vi "backup.vi"(0 "dettes":dbl, 1 "Argent ventes":dbl, 2 "CA":dbl, 3 "Impots":dbl, 4 "Calculs button":bool) -> (5 "notions_cles":dbl[](array[numeric]))   [LabVIEW 2024]
uses:
  <vilib>/express/express shared/transition.llb/Dynamic To Waveform Array.vi
  <vilib>/express/express signal manip/GetorSetDDTAttributes/Set DDT Attributes/SetT0.vi
  <vilib>/express/express shared/transition.llb/Waveform Array To Dynamic.vi
  <vilib>/express/express signal manip/GetorSetDDTAttributes/Set DDT Attributes/Set DDT Properties.xnode
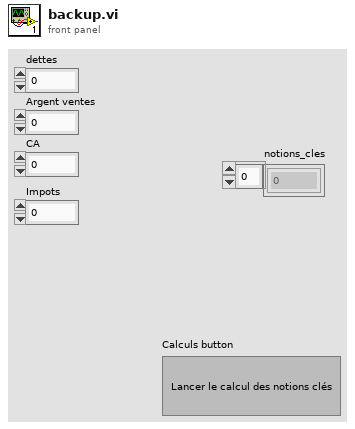
[diagram p1: front panel]
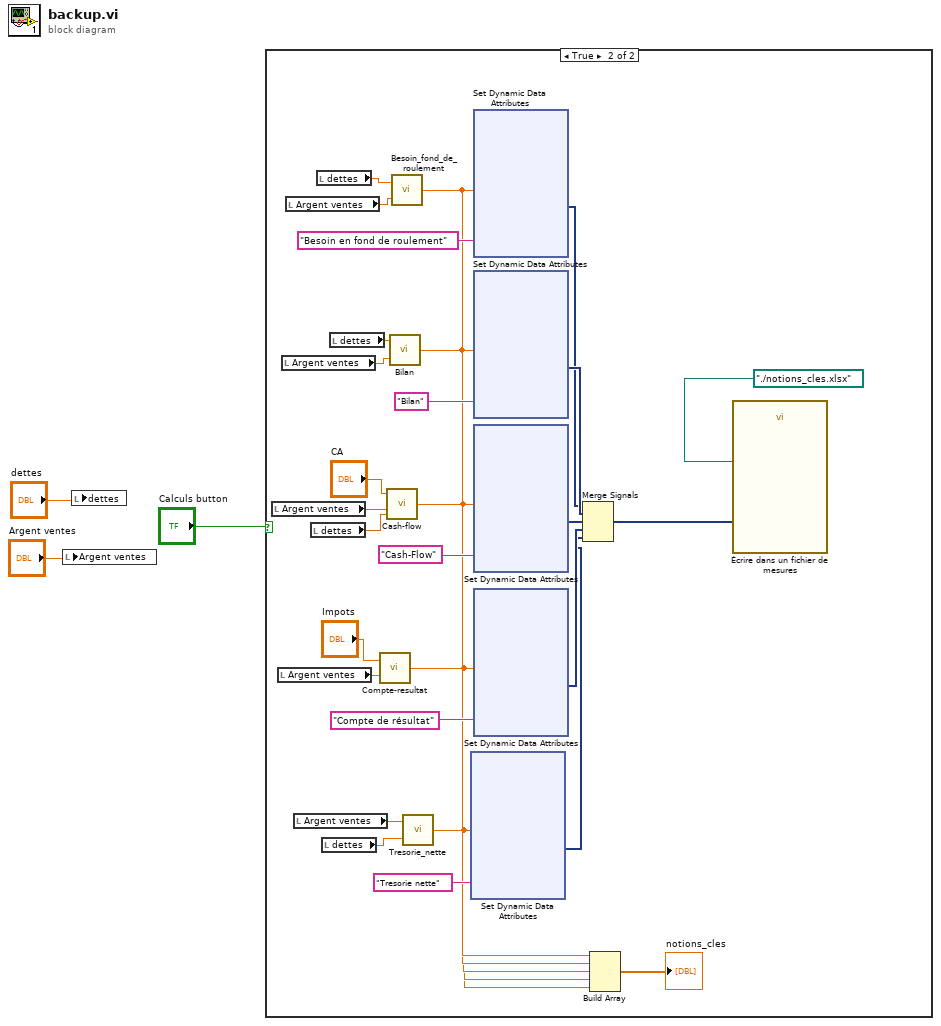
[diagram p0: block diagram]
diagram:
  n1 = local write "Argent ventes"("Argent ventes") -> ()
  n2 = local write "dettes"("dettes") -> ()
  n3 = case shown="True" "Calculs button" {
    frame False {
    }
    frame True {
      n4 = local read "Argent ventes"() -> (w16:dbl)
      n5 = local read "Argent ventes"() -> (w13:dbl)
      n6 = local read "Argent ventes"() -> (w18:dbl)
      n7 = local read "Argent ventes"() -> (w20:dbl)
      n8 = local read "Argent ventes"() -> (w12:dbl)
      n9 = local read "dettes"() -> (w15:dbl)
      n10 = local read "dettes"() -> (w21:dbl)
      n11 = local read "dettes"() -> (w11:dbl)
      n12 = local read "dettes"() -> (w19:dbl)
      n13 = call "Compte-resultat.vi"("Argent ventes"=w13, "Impots"="Impots") -> ("Compte résultat"=w5:dbl)
      n14 = call "Cash-flow.vi"("Dettes"=w15, "Argent ventes"=w16, "CA"="CA") -> ("Cash Flow"=w6:dbl)
      n15 = call "Bilan.vi"("Argent ventes"=w18, "Dettes"=w19) -> ("Bilan"=w7:dbl)
      n16 = call "Besoin_fond_de_roulement.vi"("Argent ventes"=w20, "dettes"=w21) -> ("BFR"=w8:dbl)
      n17 = call "Tresorie_nette.vi"("Dettes"=w11, "Argent ventes"=w12) -> ("tresorire nette"=w4:dbl)
      n18 = xnode "Set Dynamic Data Attributes"("Signals In"=w4, "Signal Name"="Tresorie nette") -> ("Signals Out"=w28:dynamicdata)  [unwired: 2 in, 1 out]
      n19 = xnode "Set Dynamic Data Attributes"("Signals In"=w8, "Signal Name"="Besoin en fond de roulement") -> ("Signals Out"=w27:dynamicdata)  [unwired: 2 in, 1 out]
      n20 = xnode "Set Dynamic Data Attributes"("Signals In"=w7, "Signal Name"="Bilan") -> ("Signals Out"=w31:dynamicdata)  [unwired: 2 in, 1 out]
      n21 = xnode "Set Dynamic Data Attributes"("Signals In"=w6, "Signal Name"="Cash-Flow") -> ("Signals Out"=w30:dynamicdata)  [unwired: 2 in, 1 out]
      n22 = xnode "Set Dynamic Data Attributes"("Signals In"=w5, "Signal Name"="Compte de résultat") -> ("Signals Out"=w29:dynamicdata)  [unwired: 2 in, 1 out]
      n23 = Merge Signals(w27, w31, w30, w29, w28) -> (w10:dynamicdata)
      n24 = Build Array(w8, w7, w6, w5, w4) -> (→"notions_cles":dbl[])
      n25 = call "Écrire dans un fichier de mesures"("Signals"=w10, "Filename"=path "./notions_cles.xlsx") -> ()  [unwired: 15 in, 3 out]
    }
  }
